vi "Chart Data.vi"(6 "Set Time":bool, 8 "error in (no error)":errorcluster, 9 "End":dbl, 10 "Start":dbl, 11 "HistorianCharting in":refnum<class "HistorianCharting.lvclass">) -> (0 "error out":errorcluster, 3 "HistorianCharting out":refnum<class "HistorianCharting.lvclass">)   [LabVIEW 2020, in "VolatusGUIElements.lvlib" / "HistorianCharting.lvclass"]
uses:
  HistorianCharting.lvclass
  Decimation Params.ctl
  HistorianCharting.lvclass/HistorianCharting.ctl
  Plot Time Range.vi
  Pixel Segments.vi
  Decimate Segments.vi
  First Last Samples.vi
  VolatusHistorian/Group Buffer DBL/Group Buffer DBL.lvclass
  VolatusGUIElements.lvlib
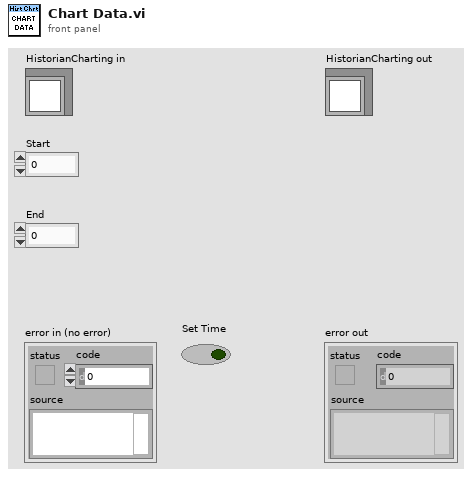
[diagram p1: front panel]
types:
  T1 = typedef "VolatusGUIElements.lvlib/Decimation Params.ctl" = cluster{"Width":i32, "Start":dbl, "End":dbl}
  T2 = typedef "VolatusGUI.lvlib/Historian Charting Manager.lvclass/X-Axis Type.ctl" = enum16{"Time", "Channel"}
  T3 = typedef "VolatusGUIElements.lvlib/HistorianCharting.lvclass/Buffer Info.ctl" = cluster{"Buffer":refnum<class "Group Buffer DBL.lvclass">, "Channels":string[], "Plot Indices":i32[]}
  T4 = typedef "VolatusHistorian.lvlib/Group Data.ctl" = cluster{"Name":string, "Timestamp":dbl[], "Channels":T5[]}
  T5 = typedef "VolatusHistorian.lvlib/Channel Data.ctl" = cluster{"Name":string, "Data":dbl[]}
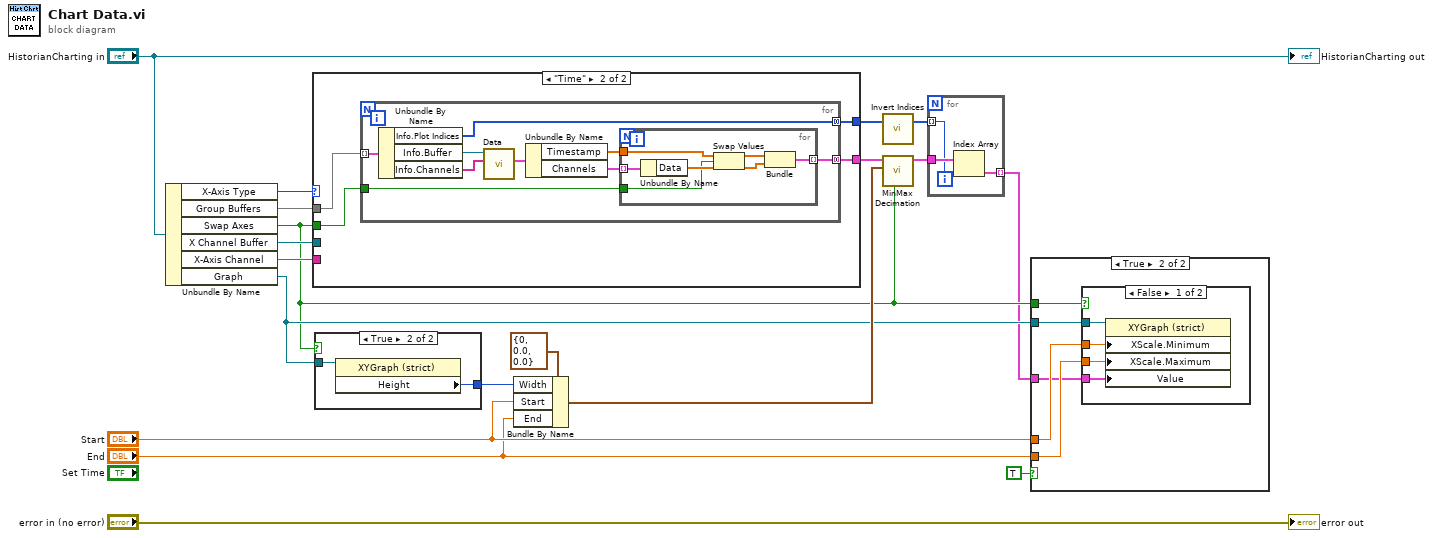
[diagram p0: block diagram]
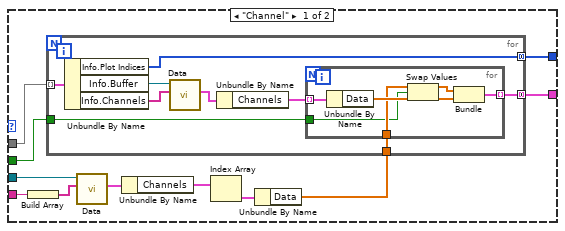
[diagram p2: hidden frame]
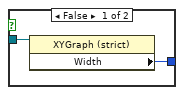
[diagram p3: hidden frame]
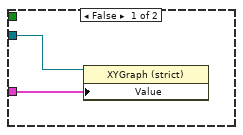
[diagram p4: hidden frame]
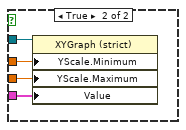
[diagram p5: hidden frame]
diagram:
  n1 = Unbundle By Name("HistorianCharting in") -> ("X-Axis Type"=w16:T2, "Group Buffers"=w17:map{string, T3}, "Swap Axes"=w6:bool, "X Channel Buffer"=w15:refnum<class "Group Buffer DBL.lvclass">, "X-Axis Channel"=w14:string, "Graph"=w9:refnum<vi>)
  n2 = case shown="\"Time\"" w16 {
    tunnel: w17 -> [w27 w50]
    tunnel: w6 -> [w26 w49]
    tunnel: w15 -> [w29 _]
    tunnel: w14 -> [w30 _]
    tunnel: [w21 w48] -> w13
    tunnel: [w20 w47] -> w4
    frame "Channel" {
      n3 = Build Array(w30) -> (w28:string[])
      n4 = call "Data.vi"("Channels (All)"=w28, "Group Buffer DBL in"=w29) -> ("Group Data"=w25:T4)  [unwired: 7 in, 2 out]
      n5 = Unbundle By Name(w25) -> ("Channels"=w24:T5[])
      n6 = Index Array(array=w24) -> (element=w23:T5)  [unwired: 1 in]
      n7 = Unbundle By Name(w23) -> ("Data"=w22:dbl[])
      n8 = for {
        tunnel: w27 -> [w39] mode=indexing
        tunnel: w26 -> [w34]
        tunnel: [w33] -> w21 mode=concatenating
        tunnel: [w32] -> w20 mode=concatenating
        tunnel: w22 -> [w31]
        n9 = Unbundle By Name(w39) -> ("Info.Plot Indices"=w32:i32[], "Info.Buffer"=w38:refnum<class "Group Buffer DBL.lvclass">, "Info.Channels"=w37:string[])
        n10 = call "Data.vi"("Channels (All)"=w37, "Group Buffer DBL in"=w38) -> ("Group Data"=w36:T4)  [unwired: 7 in, 2 out]
        n11 = Unbundle By Name(w36) -> ("Channels"=w35:T5[])
        n12 = for {
          tunnel: w35 -> [w46] mode=indexing
          tunnel: w34 -> [w40]
          tunnel: [w45] -> w33 mode=indexing
          tunnel: w31 -> [w41]
          n13 = Unbundle By Name(w46) -> ("Data"=w42:dbl[])
          n14 = Swap Values(12:w41, 13:w40, 14:w42) -> (1:w44:dbl[], 3:w43:dbl[])
          n15 = Bundle(w44, w43) -> (w45:cluster{dbl[], dbl[]})  [unwired: 1 in]
        }
      }
    }
    frame "Time" {
      n16 = for {
        tunnel: w50 -> [w59] mode=indexing
        tunnel: w49 -> [w53]
        tunnel: [w52] -> w48 mode=concatenating
        tunnel: [w51] -> w47 mode=concatenating
        n17 = Unbundle By Name(w59) -> ("Info.Plot Indices"=w51:i32[], "Info.Buffer"=w58:refnum<class "Group Buffer DBL.lvclass">, "Info.Channels"=w57:string[])
        n18 = call "Data.vi"("Channels (All)"=w57, "Group Buffer DBL in"=w58) -> ("Group Data"=w56:T4)  [unwired: 7 in, 2 out]
        n19 = Unbundle By Name(w56) -> ("Timestamp"=w55:dbl[], "Channels"=w54:T5[])
        n20 = for {
          tunnel: w55 -> [w60]
          tunnel: w54 -> [w66] mode=indexing
          tunnel: w53 -> [w63]
          tunnel: [w65] -> w52 mode=indexing
          n21 = Unbundle By Name(w66) -> ("Data"=w64:dbl[])
          n22 = Swap Values(12:w60, 13:w63, 14:w64) -> (1:w61:dbl[], 3:w62:dbl[])
          n23 = Bundle(w61, w62) -> (w65:cluster{dbl[], dbl[]})  [unwired: 1 in]
        }
      }
    }
  }
  n24 = case shown="True" w6 {
    tunnel: w9 -> [w68 w70]
    tunnel: [w67 w69] -> w10
    frame False {
      n25 = property class="XYGraph (strict)"(reference=w68) -> ("Width"=w67:u32)  [unwired: 1 in, 2 out]
    }
    frame True {
      n26 = property class="XYGraph (strict)"(reference=w70) -> ("Height"=w69:u32)  [unwired: 1 in, 2 out]
    }
  }
  n27 = Bundle By Name(cluster=T1 {"Width"=0, "Start"=0.0, "End"=0.0} ("Params"), "Width"=w10, "Start"="Start", "End"="End") -> (w11:T1)
  n28 = call "Invert Indices.vi"("Destination Indices"=w4) -> ("Source Indices"=w3:i32[])  [unwired: 6 in]
  n29 = call "MinMax Decimation.vi"("Swap Axes (F)"=w6, "Params"=w11, "XY Data"=w13) -> ("MinMax Data"=w5:cluster{dbl[], dbl[]}[])  [unwired: 8 in]
  n30 = for {
    tunnel: w5 -> [w73]
    tunnel: w3 -> [w72] mode=indexing
    tunnel: [w71] -> w2 mode=indexing
    n31 = Index Array(array=w73, index=w72) -> (element=w71:cluster{dbl[], dbl[]})
  }
  n32 = case shown="True" TRUE {
    tunnel: w9 -> [w75 w80]
    tunnel: w2 -> [w74 w77]
    tunnel: "Start" -> [_ w79]
    tunnel: "End" -> [_ w78]
    tunnel: w6 -> [_ w76]
    frame False {
      n33 = property class="XYGraph (strict)"(reference=w75, "Value"=w74) -> ()  [unwired: 1 in, 2 out]
    }
    frame True {
      n34 = case shown="False" w76 {
        tunnel: w80 -> [w84 w88]
        tunnel: w79 -> [w83 w87]
        tunnel: w78 -> [w82 w86]
        tunnel: w77 -> [w81 w85]
        frame False {
          n35 = property class="XYGraph (strict)"(reference=w84, "XScale.Minimum"=w83, "XScale.Maximum"=w82, "Value"=w81) -> ()  [unwired: 1 in, 2 out]
        }
        frame True {
          n36 = property class="XYGraph (strict)"(reference=w88, "YScale.Minimum"=w87, "YScale.Maximum"=w86, "Value"=w85) -> ()  [unwired: 1 in, 2 out]
        }
      }
    }
  }
  "error out" <- "error in (no error)"
  "HistorianCharting out" <- "HistorianCharting in"
